vi "UseThisProgramFinal.vi"() -> ()   [LabVIEW 2012]
uses:
  <vilib>/express/express analysis/Spectral/Block/exnSpectralBlock spectral measurements RMS poly.vi
  <vilib>/express/express analysis/Spectral/Block/exnSpectralBlock spectral measurements RMS DDT.vi
  <vilib>/express/express analysis/Spectral/XNode/ExpressSpectralMeasurementsBlockNode.xnode
panel:
  out "Frequency Played":dbl
  out "FFT Original":waveform(dbl)(graph)
  out "Frequency Off By":dbl
  out "Output Frequency":dbl
  out "Note Frequency":dbl
  out "Note Closest To":string
  out "Shifted Waveform":waveform(dbl)(graph)
  out "Original Waveform":dynamicdata(graph)
  # "add volume control, boolean original signal versus new, select different scales, detect when pluck string, set note frequency \nor go to closest note, fix railing, add digital effects, analog switch/potentiometer, playing a song would be awesome"
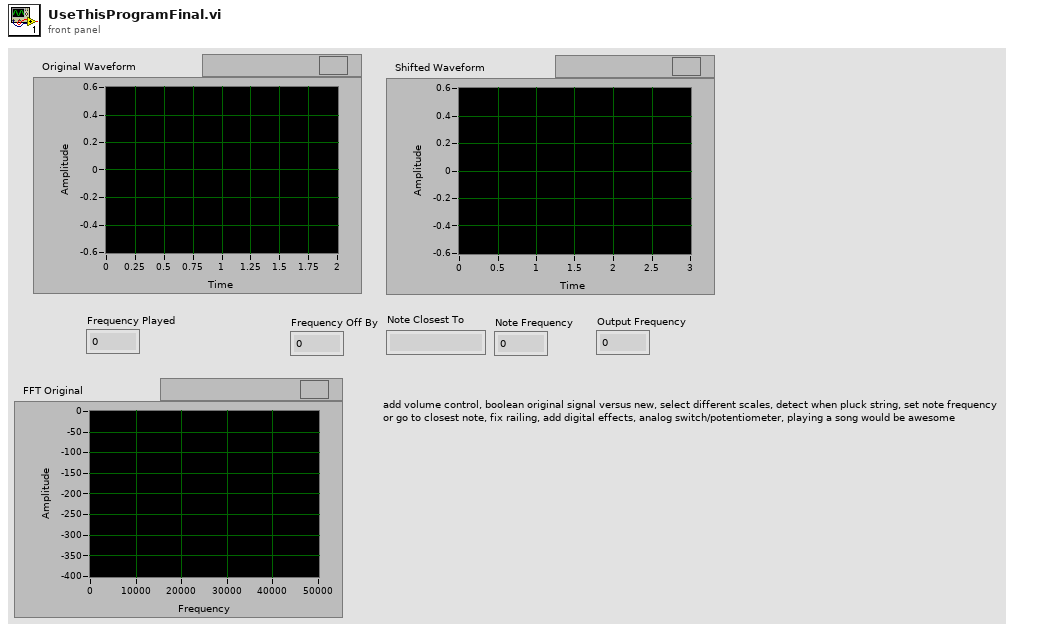
[diagram p1: front panel]
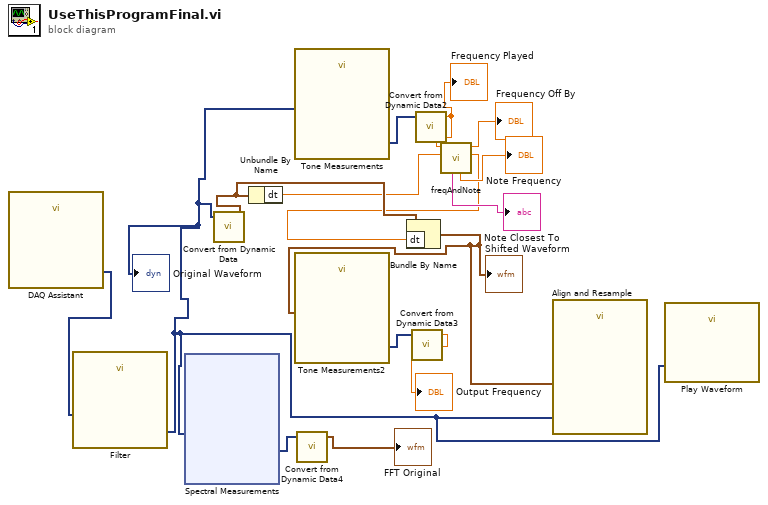
[diagram p0: block diagram]
diagram:
  n1 = call "DAQ Assistant"() -> ("data"=w14:dynamicdata)  [unwired: 17 in, 2 out]
  n2 = call "Filter"("Signal"=w14) -> ("Filtered Signal"=w15:dynamicdata)  [unwired: 9 in, 1 out]
  "Original Waveform" <- w15
  n3 = xnode "Spectral Measurements"("Signals"=w15) -> ("FFT - (RMS)"=w9:dynamicdata)  [unwired: 1 in, 2 out]
  n4 = call "Convert from Dynamic Data"("Dynamic Data Type"=w15) -> ("Waveform"=w12:waveform(dbl))  [unwired: 3 in]
  n5 = Unbundle By Name(w12) -> ("dt"=w1:dbl)
  n6 = call "Tone Measurements"("Signals"=w15) -> ("Frequency"=w2:dynamicdata)  [unwired: 8 in, 2 out]
  n7 = call "Convert from Dynamic Data4"("Dynamic Data Type"=w9) -> ("Waveform"=→"FFT Original":waveform(dbl))  [unwired: 3 in]
  n8 = call "Convert from Dynamic Data2"("Dynamic Data Type"=w2) -> ("Scalar"=w11:dbl)  [unwired: 3 in]
  "Frequency Played" <- w11
  n9 = call "freqAndNote.vi"("dt Original"=w1, "Frequency In"=w11) -> ("output dt"=w3:dbl, "Frequency Off"=→"Frequency Off By":dbl, "Note Frequency"=→"Note Frequency":dbl, "Note Closest To"=→"Note Closest To":string)  [unwired: 6 in]
  n10 = Bundle By Name(cluster=w12, "dt"=w3) -> (w13:waveform(dbl))
  "Shifted Waveform" <- w13
  n11 = call "Tone Measurements2"("Signals"=w13) -> ("Frequency"=w4:dynamicdata)  [unwired: 8 in, 2 out]
  n12 = call "Convert from Dynamic Data3"("Dynamic Data Type"=w4) -> ("Scalar"=→"Output Frequency":dbl)  [unwired: 3 in]
  n13 = call "Align and Resample"("Reference Signal"=w15, "Signals"=w13) -> ()  [unwired: 7 in, 3 out]
  n14 = call "Play Waveform"("Data"=w15) -> ()  [unwired: 18 in, 1 out]
